vi "VdTcpIP_GetAttributesToModify.vi"(0 "reference in":refnum<class "VdTcpIP.lvclass">, 3 "timeout (15000 ms)":i32=15000, 5 "error in (no error)":errorcluster) -> (14 "reference out":refnum<class "VdTcpIP.lvclass">, 16 "Attributes":T1, 17 "Timeout":bool, 19 "error out":errorcluster)   [LabVIEW 2020, in "VdTcpIP.lvclass"]
doc: "This VI returns the attributes associated with the VdSocket or subclass object reference and places a lock on the object.\n\nIf the object is currently locked for modification by another method, 'Timeout' specifies how long the VI should wait to receive access to the object. The default value waits until the object becomes available.\n\nYou must use the VdSocket SetModifiedAttributes VI to set the object's data and release the lock.\n\n[GOOP 2.0.11]"
uses:
  <instrlib>/_InstrumentDrivers/VdCommunication/VdTcpIP_class/VdTcpIP.lvclass
  <instrlib>/_InstrumentDrivers/VdCommunication/VdTcpIP_class/VdTcpIP.lvclass/VdTcpIP.ctl
  <vilib>/addons/_goop3.llb/3GOOPStates.ctl
  <instrlib>/_InstrumentDrivers/VdCommunication/VdTcpIP_class/protected/ObjectAttributes.ctl
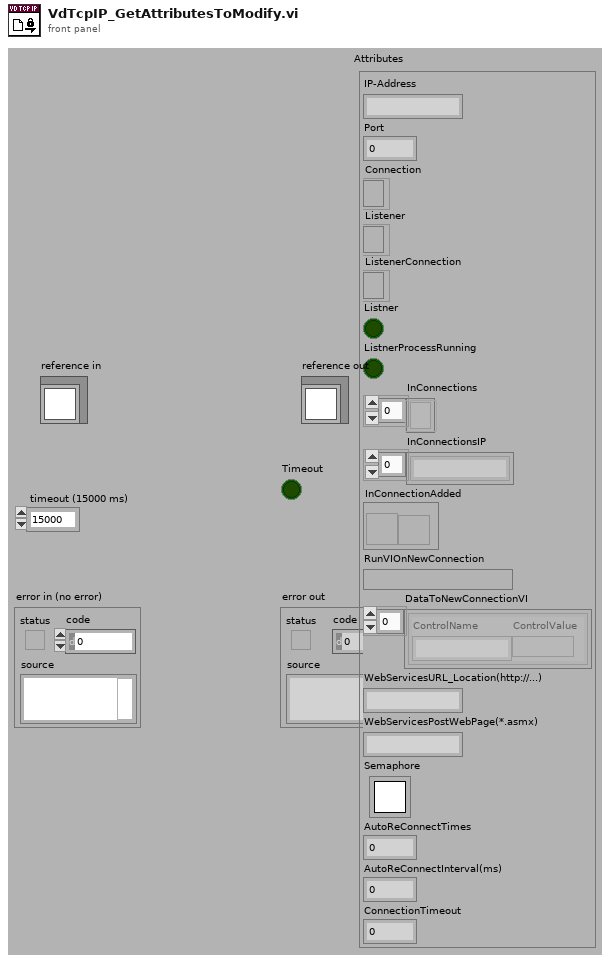
[diagram p1: front panel]
types:
  T1 = typedef "VdTcpIP.lvclass/ObjectAttributes.ctl" = cluster{"IP-Address":string, "Port":u16, "Connection":refnum<k5>, "Listener":refnum<k5>, "ListenerConnection":refnum<k5>, "Listner":bool, "ListnerProcessRunning":bool, "InConnections":refnum<k5>[], "InConnectionsIP":string[], "InConnectionAdded":refnum<notifier>, "RunVIOnNewConnection":variant, "DataToNewConnectionVI":cluster{"ControlName":string, "ControlValue":variant}[], "WebServicesURL_Location(http://...)":string, "WebServicesPostWebPage(*.asmx)":string, "Semaphore":T2, "AutoReConnectTimes":i32, "AutoReConnectInterval(ms)":i32, "ConnectionTimeout":i32}
  T2 = typedef "Semaphore RefNum" = refnum<k1>
  T3 = typedef "3GOOPStates.ctl" = enum16{"Set", "Get", "New", "Delete", "Clear", "Test and get", "Unlock data", "Information", "Look up existing", "New or look up existing", "Test and get shared", "Get shared", "Set shared", "Unlock shared", "Find dynamic method", "Register dynamic method", "Preload dynamic method", "Probe", "Cast to more generic", "Cast to more specific"}
  T4 = typedef "VdTcpIP.lvclass/ObjectReference.ctl" = refnum<k1>
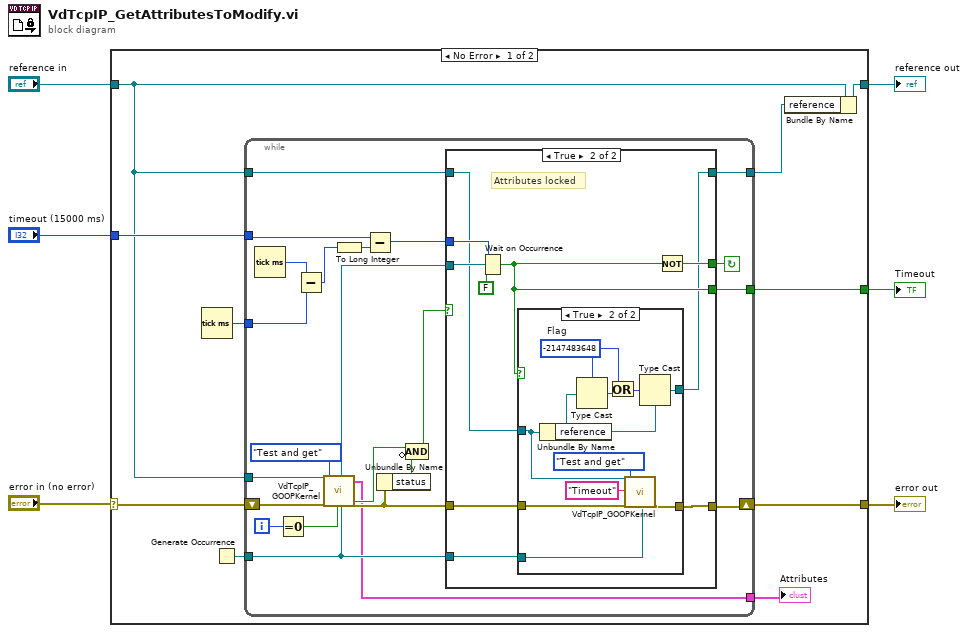
[diagram p0: block diagram]
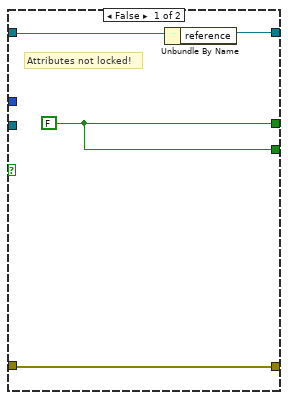
[diagram p2: hidden frame]
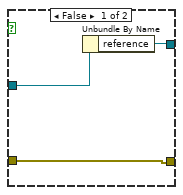
[diagram p3: hidden frame]
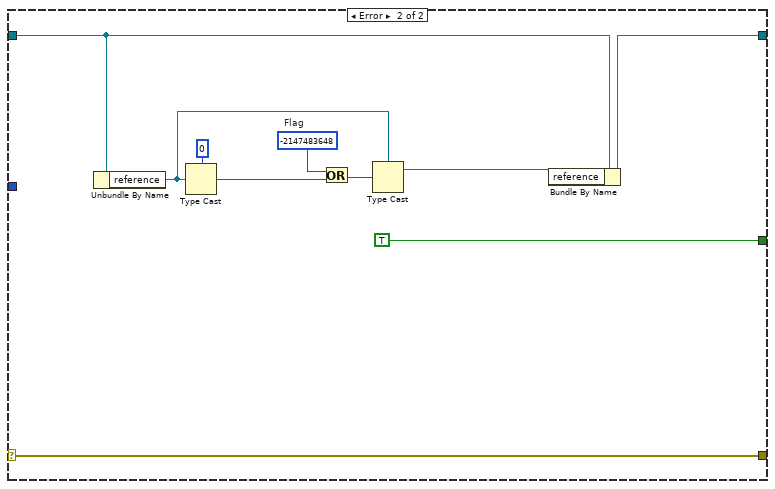
[diagram p4: hidden frame]
diagram:
  n1 = case shown="No Error" "error in (no error)" {
    selector: "error in (no error)" -> [w13 w77]
    tunnel: [w10 w73] -> w6
    tunnel: [w12 w77] -> w5
    tunnel: "reference in" -> [w8 w74]
    tunnel: [w11 TRUE ("timed out")] -> w2
    tunnel: "timeout (15000 ms)" -> [w14 _]
    frame No Error {
      n2 = Tick Count (ms)() -> (millisecond timer value=w15:u32)
      n3 = Generate Occurrence() -> (w16:refnum<k4>)
      n4 = while {
        tunnel: [w17] -> w9
        shift-left: w13 -> [w36]
        shift-right: [w22] -> w12
        tunnel: [w38] -> w11
        tunnel: w14 -> [w28]
        tunnel: w8 -> [w37]
        tunnel: w16 -> [w21]
        tunnel: w15 -> [w18]
        tunnel: w8 -> [w24]
        tunnel: [w20] -> w7
        i -> [w32]
        stop <- w39 continue-if-true
        n5 = Tick Count (ms)() -> (millisecond timer value=w19:u32)
        n6 = Equal To 0?(x=w32) -> (x = 0?=w31:bool)
        n7 = Subtract(x=w19, y=w18) -> (x-y=w27:u32)
        n8 = call <instrlib>:"VdTcpIP_GOOPKernel.vi"("Ref in"=w37, "error in (no error)"=w36, "Action"=3GOOPStates."Test and get", "Misc"=w31, "Occurrence"=w21) -> ("Occurrence out"=w30:refnum<k4>, "Data out"=w17:T1, "Data locked?"=w34:bool, "error out"=w23:errorcluster)  [unwired: 12 in, 7 out]
        n9 = To Long Integer(number=w27) -> (32bit integer=w25:i32)
        n10 = Subtract(x=w28, y=w25) -> (x-y=w26:i32)
        n11 = Unbundle By Name(w23) -> ("status"=w35:bool)
        n12 = Compound Arithmetic op=AND(w34, invert w35) -> (w33:bool)
        n13 = case shown="True" w33 {
          tunnel: w30 -> [_ w52]
          tunnel: w26 -> [_ w50]
          tunnel: [w43 w53] -> w39
          tunnel: [w43 w46] -> w38
          tunnel: w24 -> [w41 w49]
          tunnel: w23 -> [w42 w48]
          tunnel: [w42 w47] -> w22
          tunnel: w21 -> [_ w45]
          tunnel: [w40 w44] -> w20
          frame False {
            w43 = FALSE
            # "Attributes not locked!"
            n14 = Unbundle By Name(w41) -> ("reference"=w40:T4)
          }
          frame True {
            # "Attributes locked"
            n15 = Wait on Occurrence(1:FALSE ("ignore previous (T)"), 2:w52, 3:w50) -> (0:w46:bool)
            n16 = case shown="True" w46 {
              tunnel: w49 -> [w55 w61]
              tunnel: w48 -> [w56 w67]
              tunnel: [w56 w66] -> w47
              tunnel: w45 -> [_ w64]
              tunnel: [w54 w59] -> w44
              frame False {
                n17 = Unbundle By Name(w55) -> ("reference"=w54:T4)
              }
              frame True {
                w57 = -2147483648  # Flag
                n18 = Unbundle By Name(w61) -> ("reference"=w60:T4)
                n19 = Type Cast(type=w57, x=w60) -> (*(type *) &x=w62:i32)
                n20 = Or(x=w57, y=w62) -> (x .or. y?=w58:i32)
                n21 = call <instrlib>:"VdTcpIP_GOOPKernel.vi"("Ref in"=w61, "Probe in"="Timeout" ("VI ref"), "error in (no error)"=w67, "Action"=3GOOPStates."Test and get", "Occurrence"=w64) -> ("error out"=w66:errorcluster)  [unwired: 12 in, 10 out]
                n22 = Type Cast(type=w60, x=w58) -> (*(type *) &x=w59:T4)
              }
            }
            n23 = Not(x=w46) -> (.not. x?=w53:bool)
          }
        }
      }
      "Attributes" <- w9
      n24 = Bundle By Name(cluster=w8, "reference"=w7) -> (w10:refnum<class "VdTcpIP.lvclass">)
    }
    frame Error {
      w75 = -2147483648  # Flag
      n25 = Unbundle By Name(w74) -> ("reference"=w68:T4)
      n26 = Type Cast(type=0, x=w68) -> (*(type *) &x=w71:i32)
      n27 = Or(x=w75, y=w71) -> (x .or. y?=w70:i32)
      n28 = Type Cast(type=w68, x=w70) -> (*(type *) &x=w69:T4)
      n29 = Bundle By Name(cluster=w74, "reference"=w69) -> (w73:refnum<class "VdTcpIP.lvclass">)
    }
  }
  "error out" <- w5
  "reference out" <- w6
  "Timeout" <- w2
